vi "ShouldIncludeIfExternal.vi"(8 "error in (no error)":errorcluster, 9 "Current item":refnum<class "ILabVIEWItem.lvclass">, 10 "Include external?":bool, 11 "CLabVIEWItemVI in":refnum<class "CLabVIEWItemVI.lvclass">) -> (0 "error out":errorcluster, 1 "Include?":bool, 3 "CLabVIEWItemVI out":refnum<class "CLabVIEWItemVI.lvclass">)   [LabVIEW 2020, in "LabVIEWFiles.lvlib" / "CLabVIEWItemVI.lvclass"]
uses:
  CLabVIEWItemVI.lvclass
  LabVIEWObjectInterfaces/ILabVIEWItem/ILabVIEWItem.lvclass
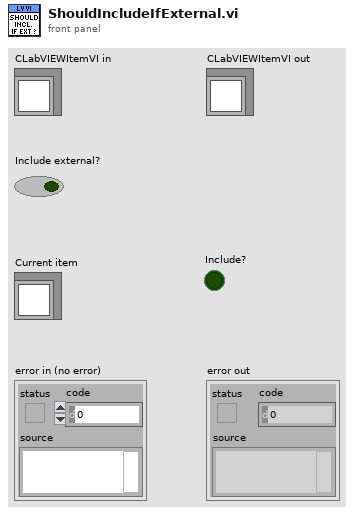
[diagram p1: front panel]
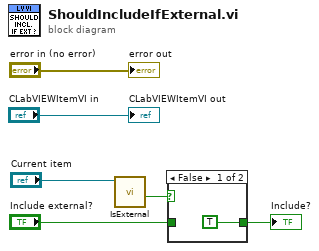
[diagram p0: block diagram]
diagram:
  n1 = call-dynamic "IsExternal.vi"("ILabVIEWItem in"="Current item") -> ("Is external?"=w6:bool)  [unwired: 8 in, 2 out]
  n2 = case shown="False" w6 {
    tunnel: [TRUE ("Include external?") w8] -> w1
    tunnel: "Include external?" -> [_ w8]
    frame False {
    }
    frame True {
    }
  }
  "Include?" <- w1
  "error out" <- "error in (no error)"
  "CLabVIEWItemVI out" <- "CLabVIEWItemVI in"
